vi "Init Pixel Array.vi"(10 "Height":i32, 11 "Width":i32) -> (3 "Pixel Array":i32[](array[numeric]))   [LabVIEW 2018]
doc: "Init the pixel buffer 1D array."
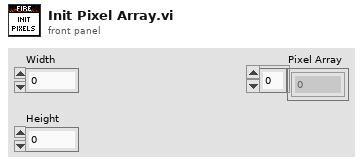
[diagram p1: front panel]
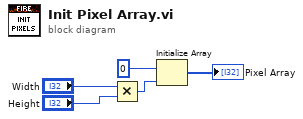
[diagram p0: block diagram]
diagram:
  n1 = Multiply(x="Width", y="Height") -> (x*y=w4:i32)
  n2 = Initialize Array(0 ("f"), w4) -> (→"Pixel Array":i32[])
